vi "Prefilter.vi"(8 "error in (no error)":errorcluster, 10 "Waveforms in":waveform(dbl)[](array[waveform]), 11 "Instrument.DAQ in":refnum<class "Instrument.DAQ.lvclass">) -> (0 "error out":errorcluster, 2 "Waveforms out":waveform(dbl)[](array[waveform]), 3 "Instrument.DAQ out":refnum<class "Instrument.DAQ.lvclass">)   [LabVIEW 2019, in "Instrument.Lockin.lvlib" / "Instrument.DAQ.lvclass"]
uses:
  Instrument.DAQ.lvclass
  Instrument.DAQ.lvclass/Instrument.DAQ.ctl
  DSP/DSP.lvclass
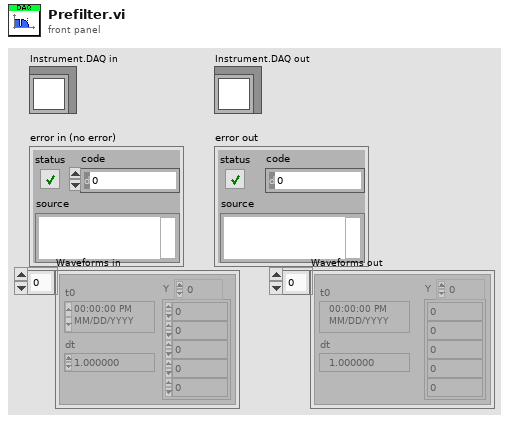
[diagram p1: front panel]
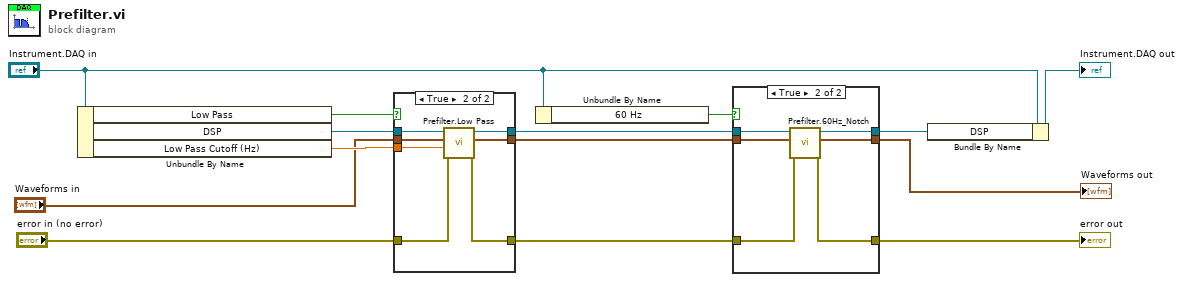
[diagram p0: block diagram]
diagram:
  n1 = Unbundle By Name("Instrument.DAQ in") -> ("Low Pass"=w5:bool, "DSP"=w7:refnum<class "DSP.lvclass">, "Low Pass Cutoff (Hz)"=w3:dbl)
  n2 = case shown="True" w5 {
    tunnel: "error in (no error)" -> [w15 w24]
    tunnel: [w17 w23] -> w12
    tunnel: [w15 w22] -> w11
    tunnel: w7 -> [w17 w21]
    tunnel: [w16 w20] -> w6
    tunnel: "Waveforms in" -> [w16 w19]
    tunnel: w3 -> [_ w18]
    frame False {
    }
    frame True {
      n3 = call "Prefilter.Low Pass.vi"("error in (no error)"=w24, "Low Pass Cutoff (Hz)"=w18, "signal in"=w19, "DSP in"=w21) -> ("error out"=w22:errorcluster, "signa out"=w20:waveform(dbl)[], "DSP out"=w23:refnum<class "DSP.lvclass">)  [unwired: 5 in]
    }
  }
  n4 = Unbundle By Name("Instrument.DAQ in") -> ("60 Hz"=w4:bool)
  n5 = case shown="True" w4 {
    tunnel: [w25 w33] -> w14
    tunnel: w12 -> [w27 w32]
    tunnel: w11 -> [w25 w31]
    tunnel: [w27 w30] -> w10
    tunnel: w6 -> [w26 w29]
    tunnel: [w26 w28] -> w2
    frame False {
    }
    frame True {
      n6 = call "Prefilter.60Hz_Notch.vi"("error in (no error)"=w31, "signal in"=w29, "DSP in"=w32) -> ("error out"=w33:errorcluster, "signal out"=w28:waveform(dbl)[], "DSP out"=w30:refnum<class "DSP.lvclass">)  [unwired: 6 in]
    }
  }
  "error out" <- w14
  "Waveforms out" <- w2
  n7 = Bundle By Name(cluster="Instrument.DAQ in", "DSP"=w10) -> (→"Instrument.DAQ out":refnum<class "Instrument.DAQ.lvclass">)
